vi "set_positioning_cursors.vi"(8 "error in (no error)":errorcluster, 11 "ColorOverlay in":refnum<class "ColorOverlay.lvclass">) -> (0 "error out":errorcluster, 3 "ColorOverlay out":refnum<class "ColorOverlay.lvclass">)   [LabVIEW 2010, in "ColorOverlay.lvclass"]
uses:
  ColorOverlay.lvclass
  ColorOverlay.lvclass/ColorOverlay.ctl
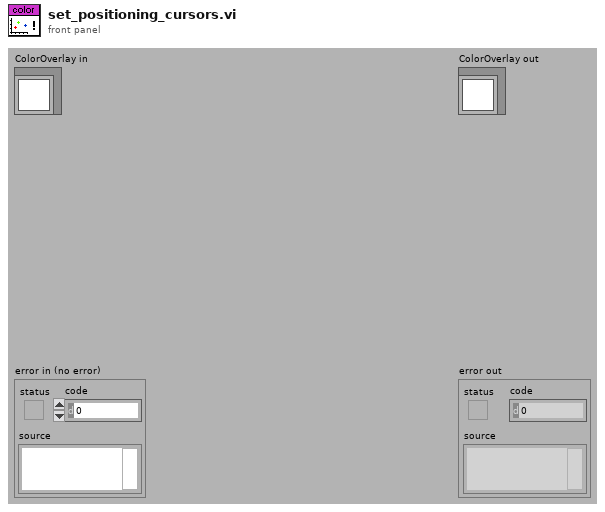
[diagram p1: front panel]
types:
  T1 = typedef "ColorOverlay.lvclass/cursor_cluster.ctl" = cluster{"cursor position":dbl[]}
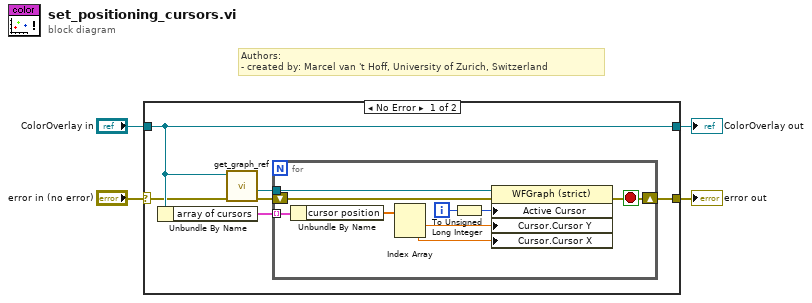
[diagram p0: block diagram]
diagram:
  # "Authors: \n- created by: Marcel van 't Hoff, University of Zurich, Switzerland"
  n1 = case shown="No Error" "error in (no error)" {
    selector: "error in (no error)" -> [w7 w21]
    tunnel: [w6 w21] -> w3
    tunnel: [w10 w20] -> w1
    tunnel: "ColorOverlay in" -> [w10 w20]
    frame No Error {
      n2 = Unbundle By Name(w10) -> ("array of cursors"=w5:T1[])
      n3 = call-dynamic "get_graph_ref.vi"("error in (no error)"=w7, "ColorOverlay in"=w10) -> ("error out"=w8:errorcluster, "graph ref"=w9:refnum<vi>)  [unwired: 7 in, 1 out]
      n4 = for {
        tunnel: w9 -> [w19]
        shift-right: [w11] -> w6
        shift-left: w8 -> [w18]
        tunnel: w5 -> [w15] mode=indexing
        i -> [w17]
        stop <- w11 stop-if-true
        n5 = Unbundle By Name(w15) -> ("cursor position"=w14:dbl[])
        n6 = Index Array(array=w14) -> (element #1=w13:dbl, element #2=w12:dbl)  [unwired: 2 in]
        n7 = To Unsigned Long Integer(number=w17) -> (unsigned 32bit integer=w16:u32)
        n8 = property class="WFGraph (strict)"(reference=w19, error in=w18, "Active Cursor"=w16, "Cursor.Cursor Y"=w13, "Cursor.Cursor X"=w12) -> (error out=w11:errorcluster)  [unwired: 1 out]
      }
    }
    frame Error {
    }
  }
  "error out" <- w3
  "ColorOverlay out" <- w1
